vi "edittest.vi"(7 "httpRequestID":u32) -> ()   [LabVIEW 2011]
doc: "This VI is a state machine that can be ran from a Browser."
uses:
  server/database/Users/User Record.ctl
  <vilib>/addons/internet/utils/strutil.llb/Case Matching.ctl
  <vilib>/wsapi/NI_WebServices.lvlib
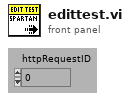
[diagram p1: front panel]
types:
  T1 = typedef "User Record.ctl" = cluster{"ixUser":i32, "sxUsername":string, "sLastName":string, "sFirstName":string, "sEmail":string, "sPassword":string, "tLoginTime":timestamp, "sLoginComputer":string, "fAdministrator":bool, "fRunSequences":bool, "fModifySequences":bool, "fRunScenarios":bool, "fModifyScenarios":bool, "fModifyTemplates":bool, "fModifyUsers":bool, "fModifyStations":bool, "fModifyFields":bool}
  T2 = typedef "Connection Refnum.ctl" = cluster{"Environment Handle":i32, "Connection Handle":i32}
  T3 = cluster{"Import? (F)":bool, "Start with Changes? (f)":bool, "Copy/Import (\"\")":string}
  T4 = typedef "Case Matching.ctl" = enum16{"a != A", "a == A", "system"}
  T5 = cluster{"Local File Path":string, "Client File Name":string, "Content Type":string, "Size":u32}[]
  T6 = typedef "Keyed Array.ctl" = cluster{"keys":string[], "values":string[]}
  T7 = typedef "Sequence Record.ctl" = cluster{"ixSequence":i32, "sxSequenceId":string, "sDescription":string, "sCreator":string, "tCreationDate":timestamp, "sModifier":string, "tModifiedDate":timestamp, "fApproved":bool, "fSpartanSetsSN":bool, "fOverwriteData":bool, "fStopOnFail":bool, "fDisableQuickMode":bool, "fPartialExecution":bool, "fAutoNextItem":bool, "fDoNotPrintOnFail":bool}
  T8 = typedef "Field Record.ctl" = cluster{"ixField":i32, "iSequenceOrder":i32, "sxFieldId":string, "sxSequenceId":string, "sDisplayName":string, "sValue":string, "sUnits":string, "nDataType":T9, "nNextItem":T10, "fSystem":bool, "fSystemValue":bool, "fRequired":bool, "fSetAtTest":bool, "fTestField":bool, "fDeleted":bool, "fIndexed":bool, "fFreeList":bool}
  T9 = typedef "Field DataTypes.ctl" = enum32{"text", "numeric", "list", "timestamp", "boolean"}
  T10 = typedef "Field NextItem.ctl" = enum32{"Reset", "Retain", "Auto-Increment"}
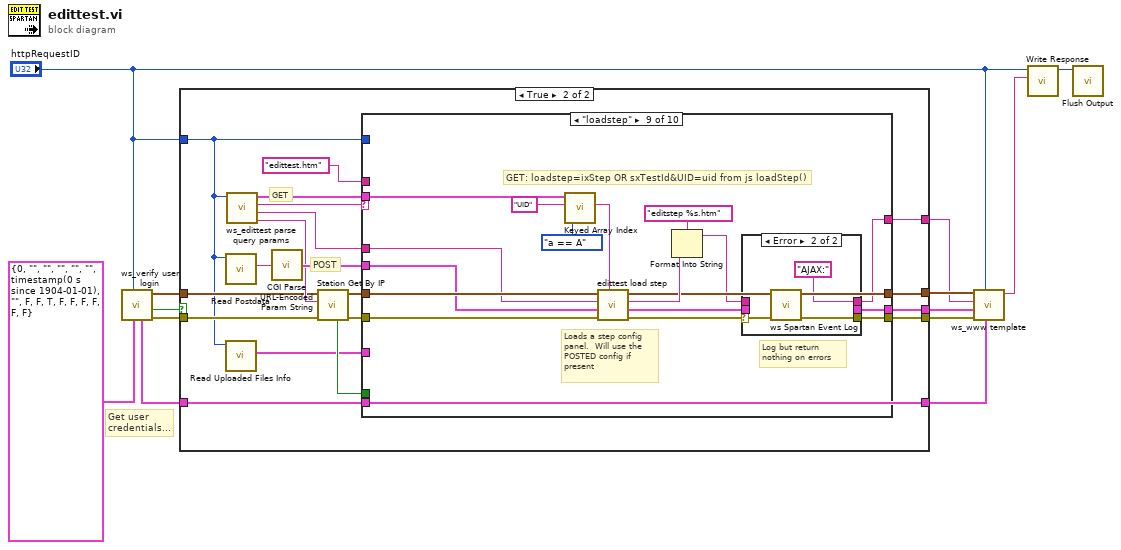
[diagram p0: block diagram]
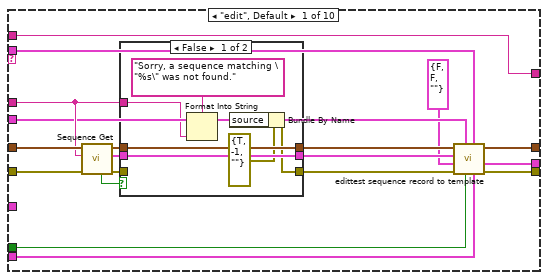
[diagram p3: hidden frame]
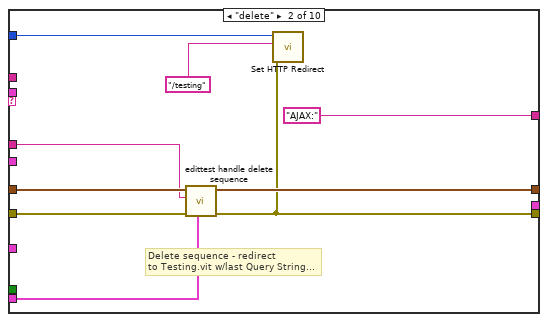
[diagram p5: hidden frame]
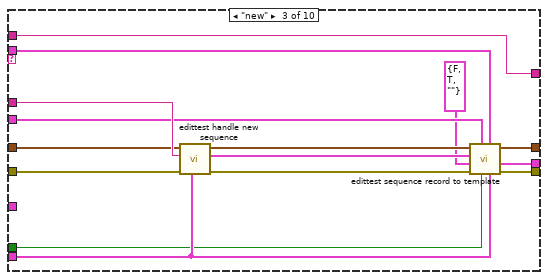
[diagram p6: hidden frame]
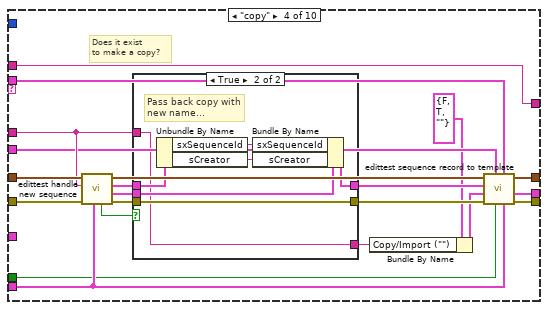
[diagram p7: hidden frame]
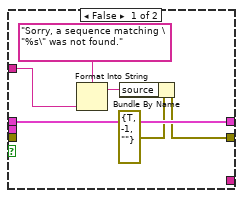
[diagram p8: hidden frame]
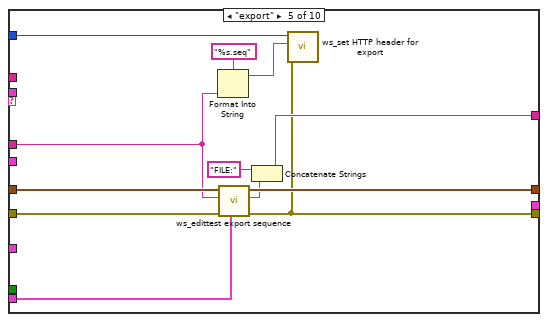
[diagram p9: hidden frame]
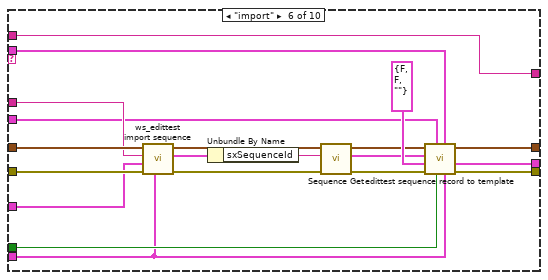
[diagram p10: hidden frame]
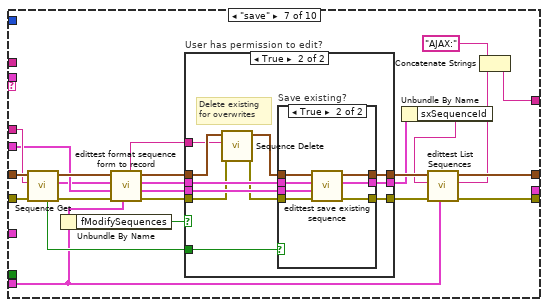
[diagram p11: hidden frame]
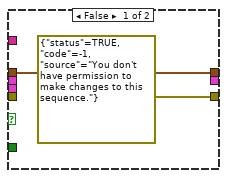
[diagram p12: hidden frame]
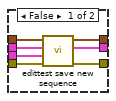
[diagram p13: hidden frame]
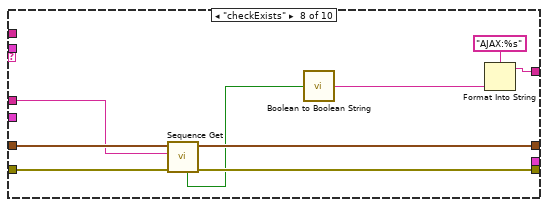
[diagram p14: hidden frame]
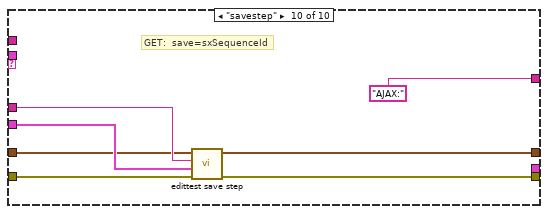
[diagram p16: hidden frame]
diagram:
  # "Get user \ncredentials..."
  n1 = call "ws_verify user login.vi"("Required Permisions"=T1 {"ixUser"=0, "sxUsername"="", "sLastName"="", "sFirstName"="", "sEmail"="", "sPassword"="", "tLoginTime"=timestamp(0 s since 1904-01-01), "sLoginComputer"="", "fAdministrator"=FALSE, "fRunSequences"=FALSE, "fModifySequences"=TRUE, "fRunScenarios"=FALSE, "fModifyScenarios"=FALSE, "fModifyTemplates"=FALSE, "fModifyUsers"=FALSE, "fModifyStations"=FALSE, "fModifyFields"=FALSE} ("User Record"), "httpRequestID"="httpRequestID") -> ("error out"=w12:errorcluster, "User Verified\nand Spartan\nAuthorized?"=w13:bool, "DB Connection Ref"=w11:T2, "User"=w9:T1)  [unwired: 6 in]
  n2 = case shown="True" w13 {
    tunnel: [w16 w26] -> w8
    tunnel: w9 -> [w14 w21]
    tunnel: w11 -> [w15 w23]
    tunnel: w12 -> [w16 w24]
    tunnel: [w15 w25] -> w7
    tunnel: [_ w20] -> w4
    tunnel: [_ w22] -> w5
    tunnel: [w14 w21] -> w6
    tunnel: "httpRequestID" -> [_ w17]
    frame False {
    }
    frame True {
      # "GET"
      # "POST"
      n3 = call <vilib>:"Read Postdata.vi"("httpRequestID"=w17) -> ("postdata"=w19:string)  [unwired: 8 in, 2 out]
      n4 = call <vilib>:"Read Uploaded Files Info.vi"("httpRequestID"=w17) -> ("UploadedFilesList"=w18:T5)  [unwired: 8 in, 2 out]
      n5 = call "ws_edittest parse query params.vi"("httpRequestID"=w17) -> ("Client Address"=w28:string, "First Value"=w32:string, "First Key"=w31:string, "Query Parameters"=w33:T6)  [unwired: 7 in]
      n6 = call <vilib>:"CGI Parse URL-Encoded Param String.vi"("url-encoded param string"=w19) -> ("params"=w34:T6)
      n7 = call "Station Get By IP.vi"("error in (no error)"=w24, "IP or Name (\"\")"=w28, "Connection Refnum"=w23) -> ("error out"=w30:errorcluster, "Connection Refnum"=w29:T2, "Data Present?"=w27:bool)  [unwired: 6 out]
      n8 = case shown="\"loadstep\"" w31 {
        tunnel: w30 -> [w52 w73 w80 w104 w134 w147 w165 w213 w223 w242]
        tunnel: w29 -> [w53 w72 w81 w106 w133 w148 w166 w214 w226 w239]
        tunnel: w32 -> [w42 w71 w84 w96 w125 w146 w164 w208 w222 w240]
        tunnel: [w54 "AJAX:" ("New URL (testing.vit)") w88 w109 w128 w150 w174 w210 w217 "AJAX:" ("key")] -> w20
        tunnel: "edittest.htm" -> [w54 _ w88 w109 _ w150 _ _ _ _]
        tunnel: [w48 w65 w86 w107 w123 w154 w178 w211 w220 w238] -> w26
        tunnel: [w49 w70 w87 w108 w131 w153 w176 w212 w224 w243] -> w25
        tunnel: w34 -> [w38 _ w76 w93 _ w138 w159 _ w215 w241]
        tunnel: [w40 _ w78 w95 _ w151 _ _ w218 _] -> w22
        tunnel: w21 -> [w41 w69 w79 w101 w132 w136 w155 _ _ _]
        tunnel: w33 -> [w39 _ w77 w94 _ w152 _ _ w225 _]
        tunnel: w27 -> [w36 _ w74 w89 _ w149 _ _ _ _]
        tunnel: w18 -> [_ _ _ _ _ w135 _ _ _ _]
        tunnel: w17 -> [_ w67 _ _ w124 _ _ _ _ _]
        frame "edit", Default {
          n9 = call "Sequence Get.vi"("error in (no error)"=w52, "sxSequenceId (\"\")"=w42, "Connection Refnum"=w53) -> ("error out"=w46:errorcluster, "Sequence Record"=w50:T7, "Connection Refnum"=w45:T2, "Data Present"=w51:bool)  [unwired: 5 out]
          n10 = case shown="False" w51 {
            tunnel: [w60 w62] -> w47
            tunnel: w50 -> [w60 w62]
            tunnel: w46 -> [_ w63]
            tunnel: w45 -> [w61 w64]
            tunnel: [w61 w64] -> w44
            tunnel: [w56 w63] -> w43
            tunnel: w42 -> [w55 _]
            frame False {
              n11 = Format Into String(format string="Sorry, a sequence matching \"%s\" was not found.", w55) -> (resulting string=w58:string)  [unwired: 2 in, 1 out]
              n12 = Bundle By Name(cluster=errorcluster {"status"=TRUE, "code"=-1, "source"=""} ("error out"), "source"=w58) -> (w56:errorcluster)
            }
            frame True {
            }
          }
          n13 = call "edittest sequence record to template.vi"("User"=w41, "REFQUERY (none)"=w39, "Test Station (F)"=w36, "POST (empty)"=w38, "error in (no error)"=w43, "Settings"=T3 {"Import? (F)"=FALSE, "Start with Changes? (f)"=FALSE, "Copy/Import (\"\")"=""}, "Sequence Record (empty)"=w47, "Connection Refnum"=w44) -> ("error out"=w48:errorcluster, "Template Keys"=w40:T6, "Connection Refnum"=w49:T2)  [unwired: 1 out]
        }
        frame "delete" {
          # "Delete sequence - redirect\nto Testing.vit w/last Query String..."
          n14 = call "edittest handle delete sequence.vi"("User Information"=w69, "error in (no error)"=w73, "Test Sequence Id (\"\")"=w71, "Connection Refnum"=w72) -> ("error out"=w65:errorcluster, "Connection Refnum"=w70:T2)  [unwired: 6 out]
          n15 = call <vilib>:"Set HTTP Redirect.vi"("error in (no error)"=w65, "redirect URL"="/testing" ("New URL (testing.vit)"), "httpRequestID"=w67) -> ()  [unwired: 7 in, 2 out]
        }
        frame "new" {
          n16 = call "edittest handle new sequence.vi"("User Information"=w79, "error in (no error)"=w80, "New Name Suggestion\n(empty - \"Username Sequence N\")"=w84, "Connection Refnum"=w81) -> ("error out"=w82:errorcluster, "New Sequence Record"=w85:T7, "Connection Refnum"=w83:T2)  [unwired: 5 out]
          n17 = call "edittest sequence record to template.vi"("User"=w79, "REFQUERY (none)"=w77, "Test Station (F)"=w74, "POST (empty)"=w76, "error in (no error)"=w82, "Settings"=T3 {"Import? (F)"=FALSE, "Start with Changes? (f)"=TRUE, "Copy/Import (\"\")"=""}, "Sequence Record (empty)"=w85, "Connection Refnum"=w83) -> ("error out"=w86:errorcluster, "Template Keys"=w78:T6, "Connection Refnum"=w87:T2)  [unwired: 1 in]
        }
        frame "copy" {
          # "Does it exist\nto make a copy?"
          n18 = call "edittest handle new sequence.vi"("User Information"=w101, "error in (no error)"=w104, "New Name Suggestion\n(empty - \"Username Sequence N\")"=w96, "Connection Refnum"=w106) -> ("error out"=w98:errorcluster, "First Matching Sequence Record"=w103:T7, "New Sequence Record"=w100:T7, "Connection Refnum"=w105:T2, "Existed?"=w99:bool)  [unwired: 3 out]
          n19 = case shown="True" w99 {
            tunnel: w103 -> [_ w122]
            tunnel: [w115 w121] -> w102
            tunnel: w100 -> [w115 w120]
            tunnel: w98 -> [_ w119]
            tunnel: [w112 w119] -> w97
            tunnel: w96 -> [w111 w118]
            tunnel: [_ w118] -> w90
            frame False {
              n20 = Format Into String(format string="Sorry, a sequence matching \"%s\" was not found.", w111) -> (resulting string=w113:string)  [unwired: 2 in, 1 out]
              n21 = Bundle By Name(cluster=errorcluster {"status"=TRUE, "code"=-1, "source"=""} ("error out"), "source"=w113) -> (w112:errorcluster)
            }
            frame True {
              # "Pass back copy with\nnew name..."
              n22 = Unbundle By Name(w120) -> ("sxSequenceId"=w117:string, "sCreator"=w116:string)
              n23 = Bundle By Name(cluster=w122, "sxSequenceId"=w117, "sCreator"=w116) -> (w121:T7)
            }
          }
          n24 = Bundle By Name(cluster=T3 {"Import? (F)"=FALSE, "Start with Changes? (f)"=TRUE, "Copy/Import (\"\")"=""} ("Settings"), "Copy/Import (\"\")"=w90) -> (w91:T3)
          n25 = call "edittest sequence record to template.vi"("User"=w101, "REFQUERY (none)"=w94, "Test Station (F)"=w89, "POST (empty)"=w93, "error in (no error)"=w97, "Settings"=w91, "Sequence Record (empty)"=w102, "Connection Refnum"=w105) -> ("error out"=w107:errorcluster, "Template Keys"=w95:T6, "Connection Refnum"=w108:T2)  [unwired: 1 in]
        }
        frame "export" {
          n26 = Format Into String(format string="%s.seq", w125) -> (resulting string=w126:string)  [unwired: 2 in, 1 out]
          n27 = call "ws_edittest export sequence.vi"("User"=w132, "error in (no error)"=w134, "Sequence ID"=w125, "Connection Refnum"=w133) -> ("error out"=w123:errorcluster, "Exported Sequence"=w129:string, "Connection Refnum"=w131:T2)  [unwired: 5 in]
          n28 = Concatenate Strings("FILE:", w129) -> (w128:string)
          n29 = call "ws_set HTTP header for export.vi"("error in (no error)"=w123, "filename (\"\")"=w126, "httpRequestID"=w124) -> ()  [unwired: 1 in, 8 out]
        }
        frame "import" {
          n30 = call "ws_edittest import sequence.vi"("User"=w136, "error in (no error)"=w147, "UploadedFilesList"=w135, "Filename"=w146, "Connection Refnum"=w148) -> ("error out"=w142:errorcluster, "Sequence Record"=w139:T7, "Connection Refnum"=w144:T2)  [unwired: 4 in]
          n31 = Unbundle By Name(w139) -> ("sxSequenceId"=w137:string)
          n32 = call "Sequence Get.vi"("error in (no error)"=w142, "sxSequenceId (\"\")"=w137, "Connection Refnum"=w144) -> ("error out"=w141:errorcluster, "Sequence Record"=w140:T7, "Connection Refnum"=w143:T2)  [unwired: 6 out]
          n33 = call "edittest sequence record to template.vi"("User"=w136, "REFQUERY (none)"=w152, "Test Station (F)"=w149, "POST (empty)"=w138, "error in (no error)"=w141, "Settings"=T3 {"Import? (F)"=FALSE, "Start with Changes? (f)"=FALSE, "Copy/Import (\"\")"=""}, "Sequence Record (empty)"=w140, "Connection Refnum"=w143) -> ("error out"=w154:errorcluster, "Template Keys"=w151:T6, "Connection Refnum"=w153:T2)  [unwired: 1 out]
        }
        frame "save" {
          n34 = call "Sequence Get.vi"("error in (no error)"=w165, "sxSequenceId (\"\")"=w164, "Connection Refnum"=w166) -> ("error out"=w170:errorcluster, "Sequence Record"=w158:T7, "Connection Refnum"=w168:T2, "Data Present"=w167:bool)  [unwired: 5 out]
          n35 = Unbundle By Name(w155) -> ("fModifySequences"=w156:bool)
          n36 = call "edittest format sequence form to record.vi"("User"=w155, "error in (no error)"=w170, "Sequence POST (empty)"=w159, "Sequence Record In"=w158, "Connection Refnum"=w168) -> ("error out"=w171:errorcluster, "Sequence Fields"=w173:T8[], "Sequence Record"=w172:T7, "dup Connection Refnum"=w169:T2, "sxSequenceId Delete"=w157:string)  [unwired: 1 in, 1 out]
          n37 = case "User has permission to edit?" shown="True" w156 {
            tunnel: w171 -> [_ w185]
            tunnel: [errorcluster {"status"=TRUE, "code"=-1, "source"="You don't have permission to make changes to this sequence."} ("error out") w190] -> w162
            tunnel: w167 -> [_ w191]
            tunnel: w169 -> [w179 w183]
            tunnel: w172 -> [_ w187]
            tunnel: w173 -> [_ w188]
            tunnel: [_ w189] -> w161
            tunnel: [w179 w186] -> w163
            tunnel: w157 -> [_ w181]
            frame False {
            }
            frame True {
              # "Delete existing\nfor overwrites"
              n38 = call "Sequence Delete.vi"("error in (no error)"=w185, "Sequence ID"=w181, "Connection Refnum"=w183) -> ("error out"=w184:errorcluster, "Connection Refnum"=w182:T2)  [unwired: 7 out]
              n39 = case "Save existing?" shown="True" w191 {
                tunnel: w184 -> [w198 w205]
                tunnel: [w197 w204] -> w190
                tunnel: [w196 w203] -> w189
                tunnel: w188 -> [w195 w200]
                tunnel: w187 -> [w194 w201]
                tunnel: w182 -> [w193 w202]
                tunnel: [w192 w199] -> w186
                frame False {
                  n40 = call "edittest save new sequence.vi"("error in (no error)"=w198, "Sequence Fields"=w195, "Sequence Record In"=w194, "Connection Refnum"=w193) -> ("error out"=w197:errorcluster, "Sequence Record"=w196:T7, "Connection Refnum"=w192:T2)  [unwired: 5 out]
                }
                frame True {
                  n41 = call "edittest save existing sequence.vi"("error in (no error)"=w205, "Sequence Fields"=w200, "Sequence Record In"=w201, "Connection Refnum"=w202) -> ("error out"=w204:errorcluster, "Sequence Record"=w203:T7, "Connection Refnum"=w199:T2)  [unwired: 1 in, 4 out]
                }
              }
            }
          }
          n42 = Unbundle By Name(w161) -> ("sxSequenceId"=w160:string)
          n43 = call "edittest List Sequences.vi"("User Information"=w155, "error in (no error)"=w162, "sxSequenceId (\"\")"=w160, "Connection Refnum"=w163) -> ("error out"=w178:errorcluster, "Sequences List"=w175:string, "Connection Refnum"=w176:T2)  [unwired: 5 out]
          n44 = Concatenate Strings("AJAX:", w175) -> (w174:string)
        }
        frame "checkExists" {
          n45 = call "Sequence Get.vi"("error in (no error)"=w213, "sxSequenceId (\"\")"=w208, "Connection Refnum"=w214) -> ("error out"=w211:errorcluster, "Connection Refnum"=w212:T2, "Data Present"=w207:bool)  [unwired: 6 out]
          n46 = call "Boolean to Boolean String.vi"("Boolean"=w207) -> ("Boolean string"=w206:string)  [unwired: 1 in]
          n47 = Format Into String(format string="AJAX:%s", w206) -> (resulting string=w210:string)  [unwired: 2 in, 1 out]
        }
        frame "loadstep" {
          # "Log but return\nnothing on errors"
          # "Loads a step config\npanel.  Will use the\nPOSTED config if\npresent"
          # "GET: loadstep=ixStep OR sxTestId&UID=uid from js loadStep()"
          n48 = call <vilib>:"Keyed Array Index.vi"("case matching (sensitive)"=Case_Matching."a == A", "key"="UID", "array in"=w225) -> ("value"=w228:string)  [unwired: 1 in, 3 out]
          n49 = call "edittest load step.vi"("incoming UID (\"\")"=w228, "error in (no error)"=w223, "POST Step Config (empty)"=w215, "sxTestId or ixStep (\"\")"=w222, "Connection Refnum"=w226) -> ("error out"=w221:errorcluster, "Template Keys"=w219:T6, "sxTestId"=w231:string, "Connection Refnum"=w224:T2)  [unwired: 3 out]
          n50 = Format Into String(format string="editstep %s.htm", w231) -> (resulting string=w216:string)  [unwired: 2 in, 1 out]
          n51 = case shown="Error" w221 {
            selector: w221 -> [w234 w236]
            tunnel: [w234 w235] -> w220
            tunnel: w219 -> [w233 _]
            tunnel: [w233 _] -> w218
            tunnel: w216 -> [w232 _]
            tunnel: [w232 "AJAX:" ("format string")] -> w217
            frame No Error {
            }
            frame Error {
              n52 = call "ws Spartan Event Log.vi"("error in (no error)"=w236) -> ("error out"=w235:errorcluster)  [unwired: 7 in]
            }
          }
        }
        frame "savestep" {
          # "GET:  save=sxSequenceId"
          n53 = call "edittest save step.vi"("error in (no error)"=w242, "POST (empty)"=w241, "sxSequenceId (\"\")"=w240, "Connection Refnum"=w239) -> ("error out"=w238:errorcluster, "Connection Refnum"=w243:T2)  [unwired: 6 out]
        }
      }
    }
  }
  n54 = call "ws_www template.vi"("User"=w6, "httpRequestID"="httpRequestID", "error in (no error)"=w8, "Template Keys (empty)"=w5, "Template (\"\")"=w4, "DB Connection Ref"=w7) -> ("HTTP Template Content"=w3:string)  [unwired: 5 in]
  n55 = call <vilib>:"Write Response.vi"("response string"=w3, "httpRequestID"="httpRequestID") -> ("httpRequestID out"=w2:u32)  [unwired: 8 in, 1 out]
  n56 = call <vilib>:"Flush Output.vi"("httpRequestID"=w2) -> ()  [unwired: 9 in, 2 out]
